vi "Configure Diode.vi"(7 "Set Aperture or NPLC? (T: Aperture)":bool, 8 "error in (no error)":errorcluster, 9 "NPLC":dbl=1.0 min=0.0005 max=15.0 step=1.0, 10 "Aperture Seconds":dbl=0.016667, 11 "VISA resource name":refnum<visa-resource-name>) -> (0 "error out":errorcluster, 3 "VISA resource name out":refnum<visa-resource-name>)   [LabVIEW 2018, in "Keithley DMM7512.lvlib"]
doc: "This VI configures the Diode measurement and the related parameters."
uses:
  <instrlib>/Keithley DMM7512/Keithley DMM7512.lvlib
panel:
  in  "Bias Level":dbl=1e-05
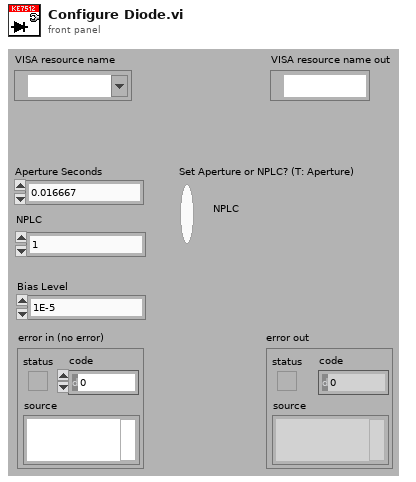
[diagram p1: front panel]
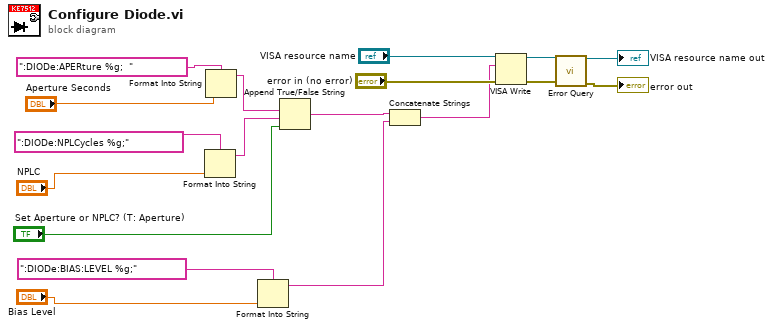
[diagram p0: block diagram]
diagram:
  n1 = Format Into String(format string=":DIODe:NPLCycles %g;", "NPLC") -> (resulting string=w3:string)  [unwired: 2 in, 1 out]
  n2 = Format Into String(format string=":DIODe:APERture %g;  ", "Aperture Seconds") -> (resulting string=w5:string)  [unwired: 2 in, 1 out]
  n3 = Format Into String(format string=":DIODe:BIAS:LEVEL %g;", "Bias Level") -> (resulting string=w1:string)  [unwired: 2 in, 1 out]
  n4 = Append True/False String(1:"Set Aperture or NPLC? (T: Aperture)", 2:w3, 3:w5) -> (0:w2:string)  [unwired: 1 in]
  n5 = Concatenate Strings(w2, w1) -> (w14:string)
  n6 = VISA Write(VISA resource name="VISA resource name", write buffer=w14, error in (no error)="error in (no error)") -> (VISA resource name out=w13:refnum<visa-resource-name>, error out=w12:errorcluster)  [unwired: 1 out]
  n7 = call <instrlib>:"Error Query.vi"("error in (no error)"=w12, "VISA resource name"=w13) -> ("error out"=→"error out":errorcluster, "VISA resource name out"=→"VISA resource name out":refnum<visa-resource-name>)  [unwired: 6 in, 2 out]
